vi "LVFunction_Imop_CameraSetupFile_GetInformationAndParamSet.vi"(0 "module path":path, 11 "error in (no error)":errorcluster) -> (4 "Camera Config":T1, 6 "AllCameraParametersProperties":T6[](array[typedef]), 15 "error out":errorcluster)   [LabVIEW 2020]
uses:
  ParameterID.ctl
  CameraParameters_Type.ctl
  CameraParameters_Authorization.ctl
  CameraParameters_OnFlyAuthorization.ctl
  CameraSpecifications.ctl
  General dimensions definition.ctl
  Point2D.ctl
  Point2Df.ctl
  Data alignment enum.ctl
  CameraSet.lvclass
  LVClass_CameraSet Read CameraParameters.vi
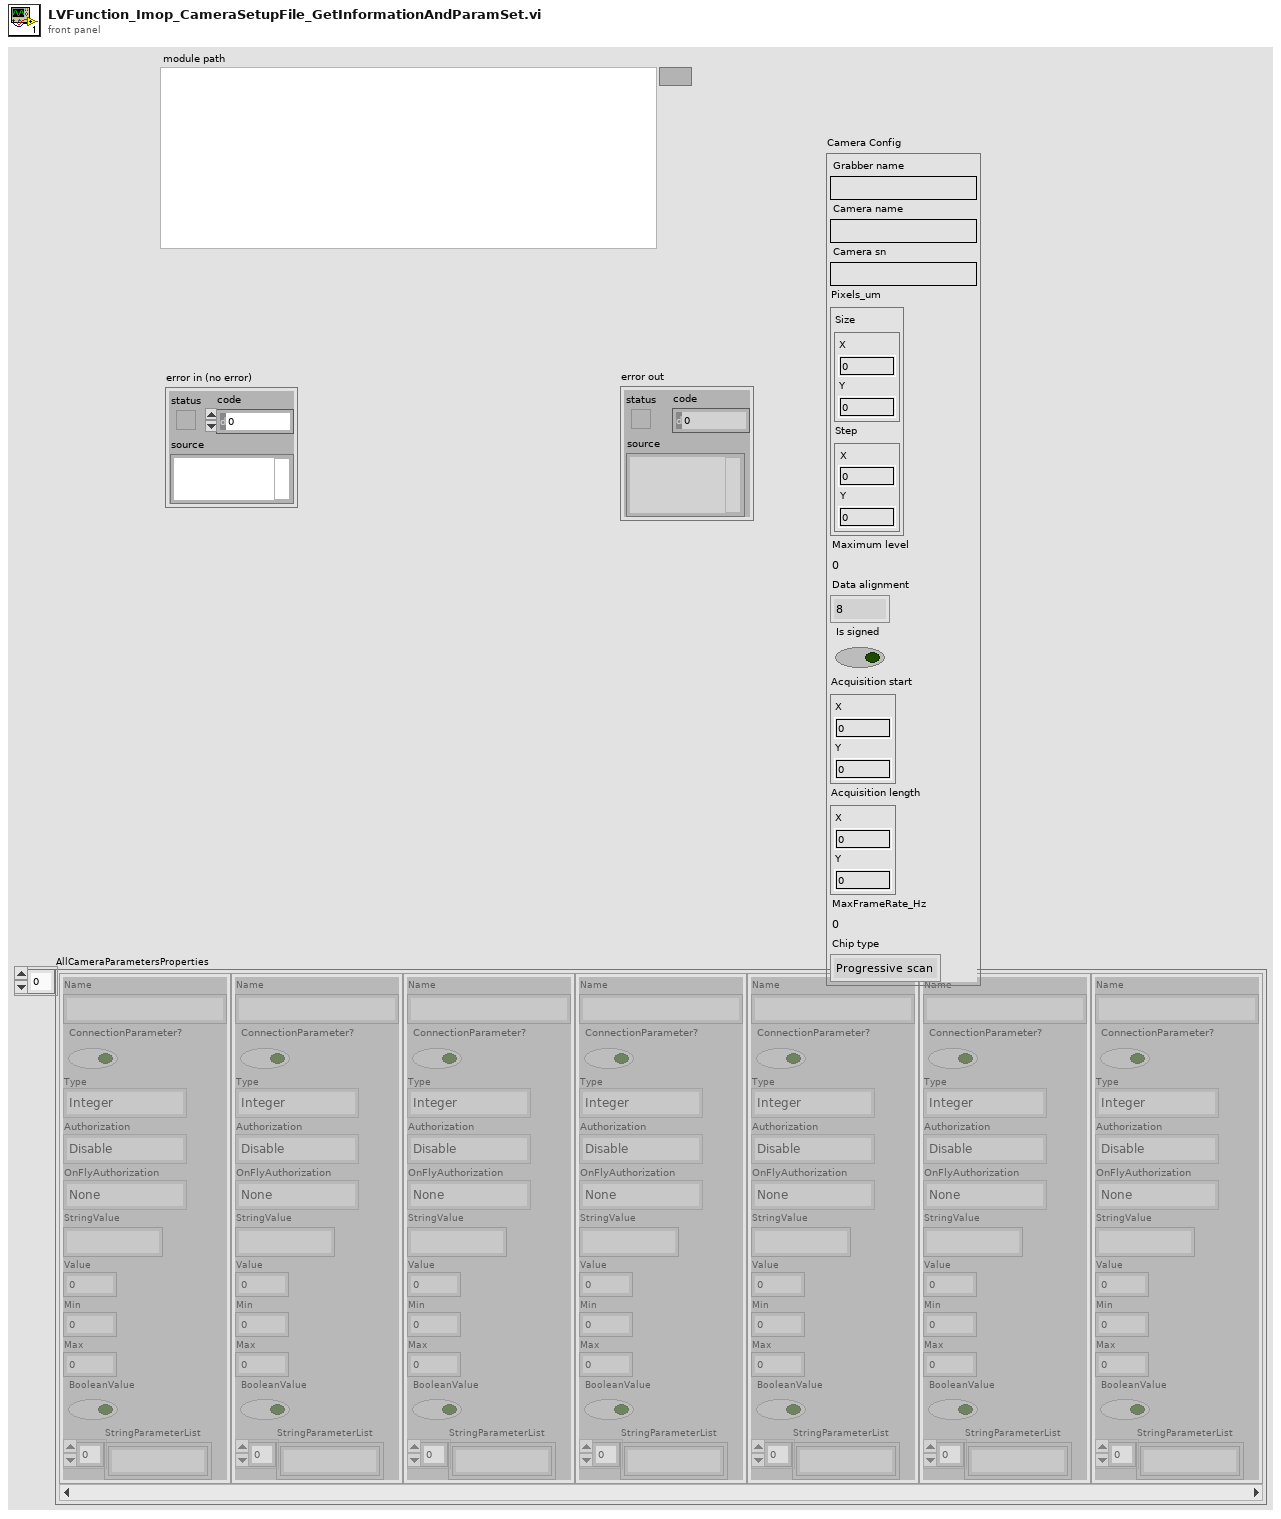
[diagram p1: front panel]
types:
  T1 = typedef "CameraSpecifications.ctl" = cluster{"Grabber name":string, "Camera name":string, "Camera sn":string, "Pixels_um":T2, "Maximum level":u32, "Data alignment":T5, "Is signed":bool, "Acquisition start":T3, "Acquisition length":T3, "MaxFrameRate_Hz":sgl, "Chip type":enum16{"Progressive scan", "Frame transfert"}}
  T2 = typedef "General dimensions definition.ctl" = cluster{"Size":T3, "Step":T4}
  T3 = typedef "Point2D.ctl" = cluster{"X":u32, "Y":u32}
  T4 = typedef "Point2Df.ctl" = cluster{"X":sgl, "Y":sgl}
  T5 = typedef "Data alignment enum.ctl" = enum16{"8", "16", "32"}
  T6 = typedef "ParameterID.ctl" = cluster{"Name":string, "ConnectionParameter?":bool, "Type":T7, "Authorization":T8, "OnFlyAuthorization":T9, "StringValue":string, "Value":dbl, "Min":dbl, "Max":dbl, "BooleanValue":bool, "StringParameterList":string[]}
  T7 = typedef "CameraParameters_Type.ctl" = enum16{"Integer", "Real", "String", "Boolean"}
  T8 = typedef "CameraParameters_Authorization.ctl" = enum16{"Disable", "Gettable", "Settable - Gettable"}
  T9 = typedef "CameraParameters_OnFlyAuthorization.ctl" = enum16{"None", "Gettable", "Settable", "Settable - Gettable"}
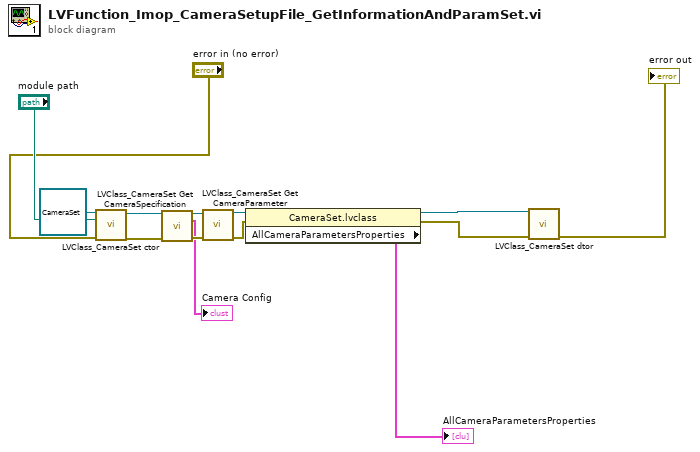
[diagram p0: block diagram]
diagram:
  n1 = call "LVClass_CameraSet ctor.vi"("CameraSet (const)"=refnum<class "CameraSet.lvclass"> refnum ("CameraSet.lvclass"), "Configuration file path"="module path", "error in (no error)"="error in (no error)") -> ("CameraSet (new)"=w7:refnum<class "CameraSet.lvclass">, "error out"=w6:errorcluster)  [unwired: 11 in]
  n2 = call "LVClass_CameraSet Get CameraSpecification.vi"("CameraSet in"=w7, "error in (no error)"=w6) -> ("CameraSet out"=w12:refnum<class "CameraSet.lvclass">, "Camera Config"=→"Camera Config":T1, "error out"=w11:errorcluster)  [unwired: 11 in]
  n3 = call "LVClass_CameraSet Get CameraParameter.vi"("CameraSet in"=w12, "error in (no error)"=w11) -> ("CameraSet out"=w14:refnum<class "CameraSet.lvclass">, "error out"=w13:errorcluster)  [unwired: 10 in, 2 out]
  n4 = property class="CameraSet.lvclass"(reference=w14, error in=w13) -> (reference out=w10:refnum<class "CameraSet.lvclass">, error out=w9:errorcluster, "AllCameraParametersProperties"=→"AllCameraParametersProperties":T6[])
  n5 = call "LVClass_CameraSet dtor.vi"("CameraSet in"=w10, "error in (no error)"=w9) -> ("error out"=→"error out":errorcluster)  [unwired: 12 in, 1 out]
